vi "Part 3 Delete From Array & Initialize Array.vi"() -> ()   [LabVIEW 2020]
panel:
  out "initialized array":dbl[](array[numeric])
  out "deleted portion":dbl
  out "array w/ subset deleted":dbl[](array[numeric])
  in  "element":dbl
  in  "array":dbl[](array[numeric])
  # "Part 3"
  # "Delete From Array & Initialize Array"
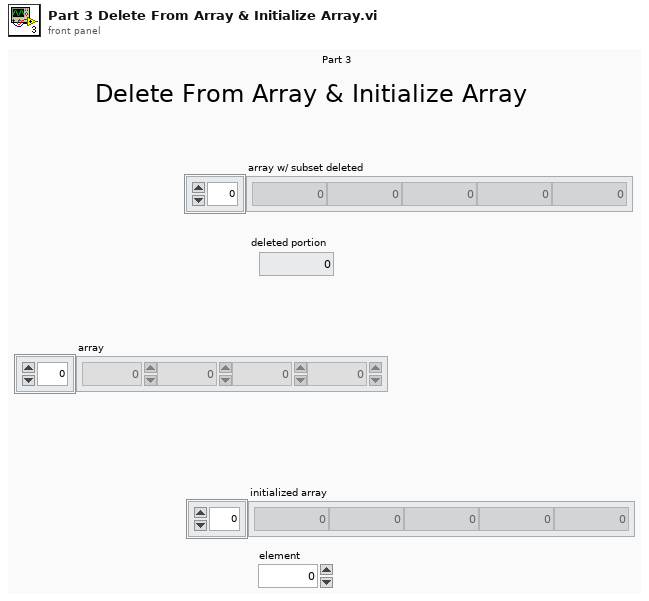
[diagram p1: front panel]
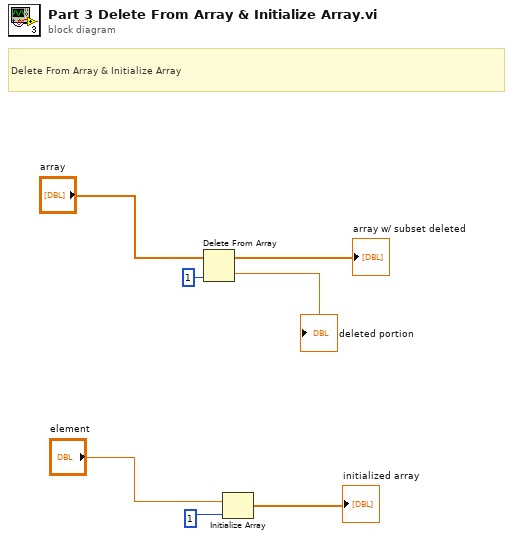
[diagram p0: block diagram]
diagram:
  # "Delete From Array & Initialize Array"
  n1 = Delete From Array "Delete From Array"(array="array", index=1) -> (deleted portion=→"deleted portion":dbl, array with subset deleted=→"array w/ subset deleted":dbl[])  [unwired: 1 in]
  n2 = Initialize Array "Initialize Array"("element", 1 ("dimension size")) -> (→"initialized array":dbl[])
